vi "Close CAN Communication.vi"(8 "error in":errorcluster, 11 "CAN Session":T1) -> (0 "error out":errorcluster)   [LabVIEW 2016]
doc: "This VI closes all memory and reference associated with the CAN communication thread."
uses:
  Low Level VIs/Typedefs/CAN Refnum.ctl
  Low Level VIs/Typedefs/CAN Session Pointer.ctl
  Low Level VIs/Typedefs/CAN Communication References.ctl
  Low Level VIs/Typedefs/kill process notifier array.ctl
  Low Level VIs/Typedefs/Write Queue.ctl
  Low Level VIs/Typedefs/FPGA CAN Frame Cluster.ctl
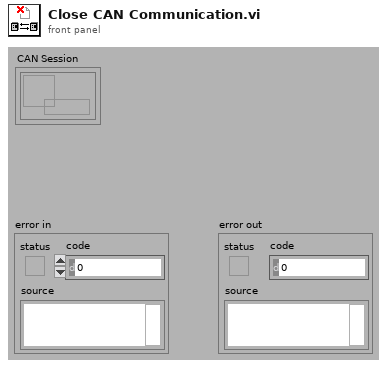
[diagram p1: front panel]
types:
  T1 = typedef "CAN Refnum.ctl" = refnum<k1>
  T2 = typedef "kill process notifier array.ctl" = refnum<notifier>[]
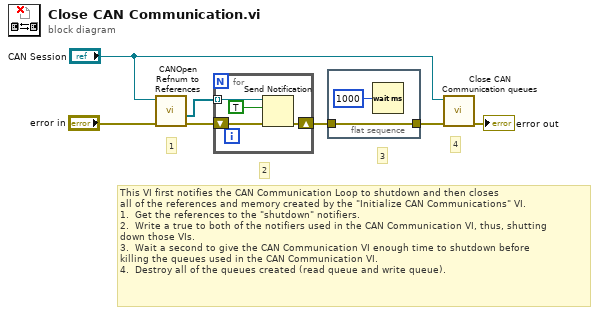
[diagram p0: block diagram]
diagram:
  # "4"
  # "3"
  # "2"
  # "1"
  # "This VI first notifies the CAN Communication Loop to shutdown and then closes\nall of the references and memory created by the \"Initialize CAN Communications\" VI. \n1.  Get the references to the \"shutdown\" notifiers.\n2.  Write a true to both of the notifiers used in the CAN Communication VI, thus, shutting\ndown those VIs.\n3.  Wait a second to give the CAN Communication VI enough time to shutdown before\nkilling the queues used in the CAN Communication VI.\n4.  Destroy all of the queues created (read queue and write queue)."
  n1 = call "CANOpen Refnum to References.vi"("error in (no error)"="error in", "CAN Session In"="CAN Session") -> ("error out"=w6:errorcluster, "kill process notifier array"=w5:T2)  [unwired: 8 out]
  n2 = for {
    shift-right: [w10] -> w4
    shift-left: w6 -> [w11]
    tunnel: w5 -> [w8] mode=indexing
    n3 = Send Notification(notification=TRUE, notifier=w8, error in (no error)=w11) -> (error out=w10:errorcluster)  [unwired: 1 out]
  }
  n4 = flat-sequence {
    tunnel: w4 -> [w13]
    tunnel: [w13] -> w3
    frame #0 {
      n5 = Wait (ms)(milliseconds to wait=u32 1000) -> ()  [unwired: 1 out]
    }
  }
  n6 = call "Close CAN Communication queues.vi"("error in"=w3, "CAN Session In"="CAN Session") -> ("error out"=→"error out":errorcluster)  [unwired: 2 in, 7 out]
